vi "ProjectileFINAL.vi"() -> ()   [LabVIEW 2014]
uses:
  <vilib>/imath/engines/lvmath2/RunTimeEngine/Managers/WorkSpace/UID Generator.vi
  <vilib>/imath/engines/lvmath2/RunTimeEngine/RunTimeType/NIMS_RunTimeType_From StrictType (excl LVString).vi
  <instcachedir>/0/NIMS_RunTimeType_From StrictType (excl LVString)_6F30FCEAD152B34FB6BC3D48AAFE00E6.lvgen/NIMS_RunTimeType_From StrictType (excl LVString)_6F30FCEAD152B34FB6BC3D48AAFE00E6_000.vi
  <vilib>/imath/engines/lvmath2/RunTimeEngine/LocalVariableDefStatement/MC_LocalVariableDefStatement_Display.vi
  <vilib>/imath/engines/lvmath2/RunTimeEngine/ArithmeticOperatorToken/NIMS_ArithmeticOperator_power(S).vi
  <instcachedir>/0/NIMS_ArithmeticOperator_power(S)_7E7603DDFF3F9240B7D001B368291B9B.lvgen/NIMS_ArithmeticOperator_power(S)_7E7603DDFF3F9240B7D001B368291B9B_014.vi
  <vilib>/imathl/engines/lvmath/Functions/Error Handling/Create Error.vi
  <vilib>/imath/engines/lvmath2/RunTimeEngine/Managers/SymbolTable/Clear UID.vi
  <vilib>/imath/engines/lvmath2/RunTimeEngine/NodeEndStatement/NIMS_NodeEndStatement_Output.vi
  <instcachedir>/0/NIMS_NodeEndStatement_Output_53EC0D466D134D7ABD903AC30B43404B.lvgen/NIMS_NodeEndStatement_Output_53EC0D466D134D7ABD903AC30B43404B_005.vi
  <instcachedir>/0/NIMS_NodeEndStatement_Output_53EC0D466D134D7ABD903AC30B43404B.lvgen/NIMS_NodeEndStatement_Output_53EC0D466D134D7ABD903AC30B43404B_004.vi
  <vilib>/imath/engines/lvmath2/RunTimeEngine/ErrorHandling/NIMS_Finalize Error.vi
  <vilib>/imath/engines/lvmath2/RunTimeEngine/Managers/SymbolTable/NIMS_WorkSpace.lvlib
panel:
  in  "Launch Parameters":T1
  out "XY Graph":cluster{"theta":i32[], "R":dbl[]}(graph)
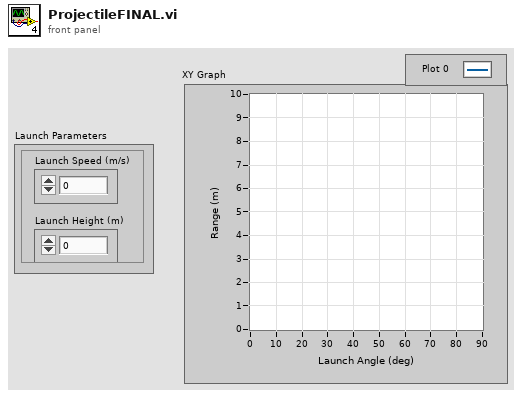
[diagram p1: front panel]
types:
  T1 = cluster{"Launch Height (m)":dbl, "Launch Speed (m/s)":dbl}
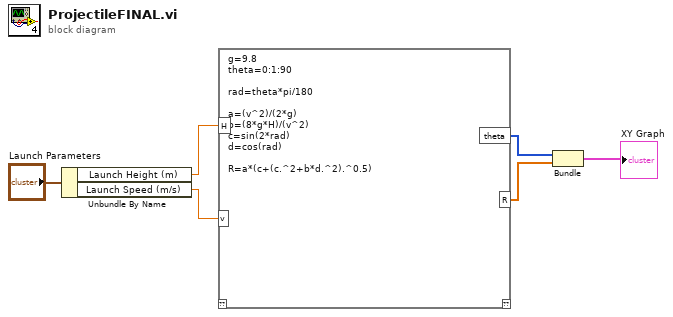
[diagram p0: block diagram]
diagram:
  n1 = Unbundle By Name("Launch Parameters") -> ("Launch Height (m)"=w5:dbl, "Launch Speed (m/s)"=w4:dbl)
  n2 = mathscript code="g=9.8\ntheta=0:1:90\n\nrad=theta*pi/180\n\na=(v^2)/(2*g)\nb=(8*g*H)/(v^2)\nc=sin(2*rad)\nd=cos(rad)\n\nR=a*(c+(c.^2+b*d.^2).^0.5)"("v"=w4, "H"=w5) -> ("theta"=w3:i32[], "R"=w2:dbl[])  [unwired: 1 in, 1 out]
  n3 = Bundle("theta"=w3, "R"=w2) -> (→"XY Graph":cluster{"theta":i32[], "R":dbl[]})  [unwired: 1 in]
